vi "GetRawDataFilePaths.vi"(8 "Force Fresh File Read?":bool, 11 "Results file or Folder":path) -> (3 "RawDataFilePaths":string[](array[string]))   [LabVIEW 2021]
uses:
  0437a104-aefb-144f-b0db-89e4e0da6f1c.vi
  Globals/Constants_global.vi
  <vilib>/Utility/file.llb/Read Delimited Spreadsheet (string).vi
panel:
  out "time(s)":dbl
  out "TPTreadGood?":bool
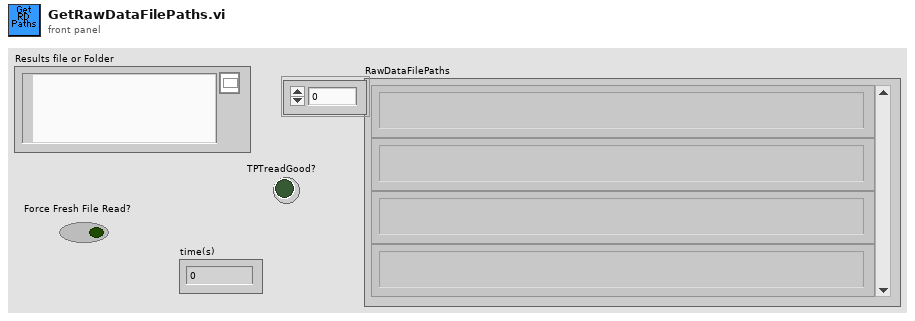
[diagram p1: front panel]
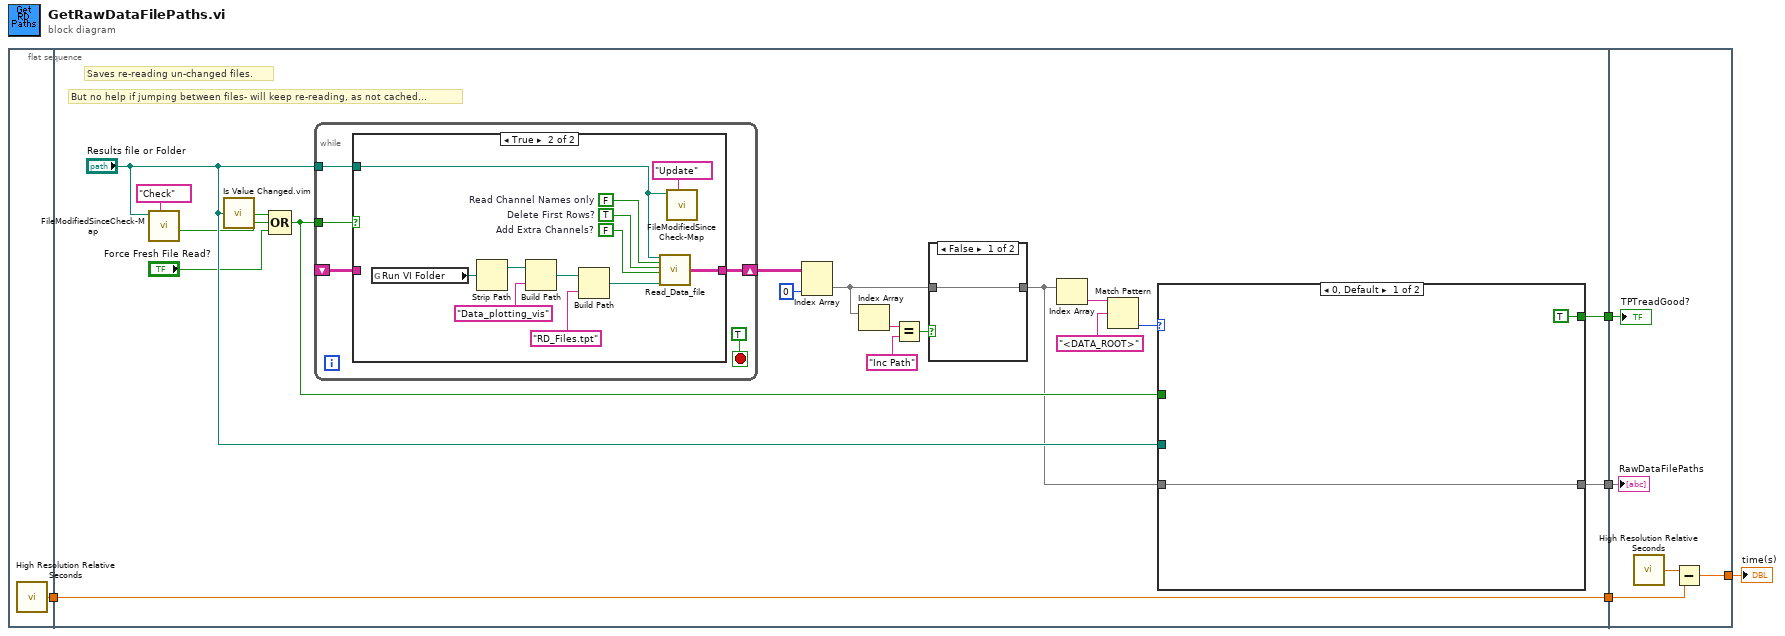
[diagram p0: block diagram]
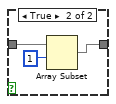
[diagram p3: hidden frame]
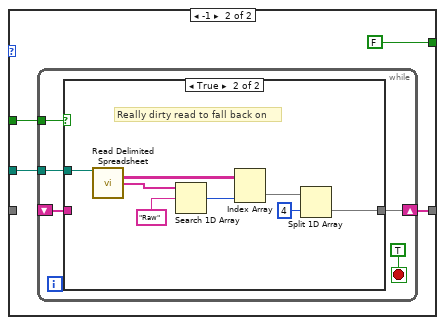
[diagram p4: hidden frame]
diagram:
  n1 = flat-sequence {
    tunnel: [w6] -> w2
    tunnel: [w10] -> w5
    tunnel: [w9] -> w4
    tunnel: [w8] -> w3
    tunnel: w2 -> [w8]
    tunnel: w5 -> [w72]
    tunnel: w4 -> [w71]
    tunnel: w3 -> [w69]
    tunnel: [w68] -> w1
    frame #0 {
      n2 = call <vilib>:"High Resolution Relative Seconds.vi"() -> ("relative seconds"=w6:dbl)
    }
    frame #1 {
      # "But no help if jumping between files- will keep re-reading, as not cached..."
      # "Saves re-reading un-changed files."
      n3 = call "FileModifiedSinceCheck-Map.vi"("mode"="Check", "file"="Results file or Folder") -> ("changed?"=w15:bool)  [unwired: 8 in, 1 out]
      n4 = call "Is Value Changed.vim"("value"="Results file or Folder") -> ("changed or first call?"=w7:bool)
      n5 = Compound Arithmetic op=OR(w7, w15, "Force Fresh File Read?") -> (w13:bool)
      n6 = while {
        shift-right: [w30] -> w25
        shift-left: _ -> [w29]
        tunnel: "Results file or Folder" -> [w27]
        tunnel: w13 -> [w26]
        stop <- TRUE stop-if-true
        n7 = case shown="True" w26 {
          tunnel: [w31 w34] -> w30
          tunnel: w29 -> [w31 _]
          tunnel: w27 -> [_ w33]
          frame False {
          }
          frame True {
            w35 = TRUE  # Delete First Rows?
            w43 = FALSE  # Add Extra Channels?
            w42 = FALSE  # Read Channel Names only
            n8 = global read "Constants_global.vi" "Run VI Folder"() -> (w39:path)
            n9 = Strip Path(path=w39) -> (stripped path=w38:path)  [unwired: 1 out]
            n10 = Build Path(base path=w38, name or relative path="Data_plotting_vis") -> (appended path=w37:path)
            n11 = Build Path(base path=w37, name or relative path="RD_Files.tpt") -> (appended path=w41:path)
            n12 = call "Read_Data_file.vi"("Results file"=w33, "Read Channel Names only"=w42, "Delete First Rows?"=w35, "Add Extra Channels?"=w43, "Template File"=w41) -> ("Channel Values Out"=w34:string[][])  [unwired: 2 in, 12 out]
            n13 = call "FileModifiedSinceCheck-Map.vi"("mode"="Update", "file"=w33) -> ()  [unwired: 8 in, 2 out]
          }
        }
      }
      n14 = Index Array(array=w25, index (col)=0 ("disabled index (col)")) -> (element=w20:string[])  [unwired: 1 in]
      n15 = Index Array(array=w20) -> (element=w21:string)  [unwired: 1 in]
      n16 = Equal?(x=w21, y="Inc Path") -> (x = y?=w23:bool)
      n17 = case shown="False" w23 {
        tunnel: w20 -> [w44 w47]
        tunnel: [w44 w45] -> w11
        frame False {
        }
        frame True {
          n18 = Array Subset(array=w47, index=1) -> (w45:string[])  [unwired: 1 in]
        }
      }
      n19 = Index Array(array=w11) -> (element=w19:string)  [unwired: 1 in]
      n20 = Match Pattern(string=w19, regular expression="<DATA_ROOT>") -> (offset past match=w12:i32)  [unwired: 1 in, 3 out]
      n21 = case shown="0, Default" w12 {
        tunnel: "Results file or Folder" -> [_ w53]
        tunnel: w13 -> [_ w52]
        tunnel: [w49 w51] -> w10
        tunnel: w11 -> [w49 _]
        tunnel: [TRUE FALSE] -> w9
        frame 0, Default {
        }
        frame -1 {
          n22 = while {
            tunnel: w53 -> [w58]
            shift-right: [w57] -> w51
            shift-left: _ -> [w56]
            tunnel: w52 -> [w54]
            stop <- TRUE stop-if-true
            n23 = case shown="True" w54 {
              tunnel: w58 -> [_ w67]
              tunnel: [w59 w60] -> w57
              tunnel: w56 -> [w59 _]
              frame False {
              }
              frame True {
                # "Really dirty read to fall back on"
                n24 = call-poly <vilib>:"Read Delimited Spreadsheet.vi"("file path (dialog if empty)"=w67) -> ("all rows"=w64:string[][], "first row"=w66:string[])  [unwired: 9 in, 4 out]
                n25 = Search 1D Array(1D array=w66, element="Raw") -> (index of element=w63:i32)  [unwired: 1 in]
                n26 = Index Array(array=w64, index (col)=w63) -> (element=w62:string[])  [unwired: 1 in]
                n27 = Split 1D Array(array=w62, index=4) -> (second subarray=w60:string[])  [unwired: 1 out]
              }
            }
          }
        }
      }
    }
    frame #2 {
      n28 = call <vilib>:"High Resolution Relative Seconds.vi"() -> ("relative seconds"=w70:dbl)
      n29 = Subtract(x=w70, y=w69) -> (x-y=w68:dbl)
      "RawDataFilePaths" <- w72
      "TPTreadGood?" <- w71
    }
  }
  "time(s)" <- w1
